vi "LS330_ArrayCul.vi"(9 "Max Size":i32, 10 "Cluster Array IN":T1) -> (2 "output cluster":T1)   [LabVIEW 2021]
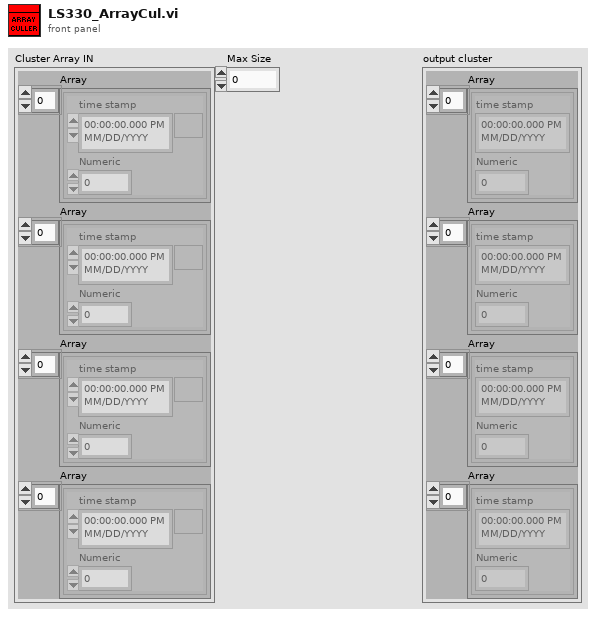
[diagram p1: front panel]
types:
  T1 = cluster{"Array":cluster{"time stamp":timestamp, "Numeric":dbl}[], "Array":cluster{"time stamp":timestamp, "Numeric":dbl}[], "Array":cluster{"time stamp":timestamp, "Numeric":dbl}[], "Array":cluster{"time stamp":timestamp, "Numeric":dbl}[]}
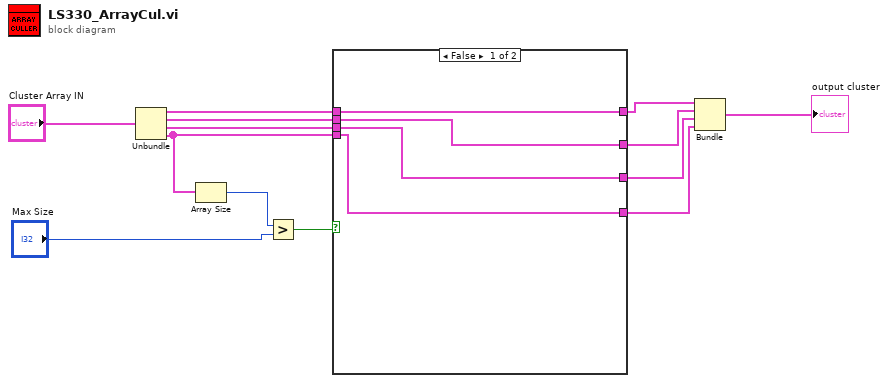
[diagram p0: block diagram]
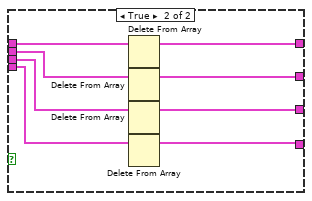
[diagram p2: hidden frame]
diagram:
  n1 = Unbundle("Cluster Array IN") -> ("Array"=w6:cluster{"time stamp":timestamp, "Numeric":dbl}[], "Array"=w7:cluster{"time stamp":timestamp, "Numeric":dbl}[], "Array"=w8:cluster{"time stamp":timestamp, "Numeric":dbl}[], "Array"=w9:cluster{"time stamp":timestamp, "Numeric":dbl}[])
  n2 = Array Size(array=w9) -> (size(s)=w11:i32)
  n3 = Greater?(x=w11, y="Max Size") -> (0:w10:bool)
  n4 = case shown="False" w10 {
    tunnel: w9 -> [w14 w22]
    tunnel: w8 -> [w15 w23]
    tunnel: w7 -> [w16 w24]
    tunnel: w6 -> [w17 w25]
    tunnel: [w17 w21] -> w5
    tunnel: [w16 w20] -> w4
    tunnel: [w15 w19] -> w3
    tunnel: [w14 w18] -> w2
    frame False {
    }
    frame True {
      n5 = Delete From Array(array=w25) -> (array with subset deleted=w21:cluster{"time stamp":timestamp, "Numeric":dbl}[])  [unwired: 2 in, 1 out]
      n6 = Delete From Array(array=w24) -> (array with subset deleted=w20:cluster{"time stamp":timestamp, "Numeric":dbl}[])  [unwired: 2 in, 1 out]
      n7 = Delete From Array(array=w23) -> (array with subset deleted=w19:cluster{"time stamp":timestamp, "Numeric":dbl}[])  [unwired: 2 in, 1 out]
      n8 = Delete From Array(array=w22) -> (array with subset deleted=w18:cluster{"time stamp":timestamp, "Numeric":dbl}[])  [unwired: 2 in, 1 out]
    }
  }
  n9 = Bundle("Array"=w5, "Array"=w4, "Array"=w3, "Array"=w2) -> (→"output cluster":T1)  [unwired: 1 in]
